vi "KE622x -- 2182 -A Get Params.vi"(0 "622x Resource In":refnum<visa-resource-name>, 1 "Check For SCPI Errors? (T)":bool=TRUE, 11 "error in (no error)":errorcluster) -> (4 "622x Resource Out (dupl)":refnum<visa-resource-name>, 8 "2182 -A Params":T1={"Auto Range?"=FALSE, "Man / Selected\n        Range"=0, "Enable Digital\n       Filter?"=FALSE, "Filter Type"=0, "Filter Count"=1, "      Filter\nWindow (%)"=0.01, "Enable Analog\n       Filter?"=FALSE, "NPLCs"=5} {"NPLCs" min=1 max=10; "Filter\nWindow (%)" min=0.01 max=10.0 step=0.01 format="%.2f"; "Filter Count" min=1 max=100; "Filter Type" items=["Movin", "Repeat"]; "Man / Selected\n        Range" items=["10mV", "100mV", "1V", "10V", "100V"]}, 15 "error out":errorcluster)   [LabVIEW 2013, in "Keithly user program.lvlib"]
uses:
  Keithly user program.lvlib
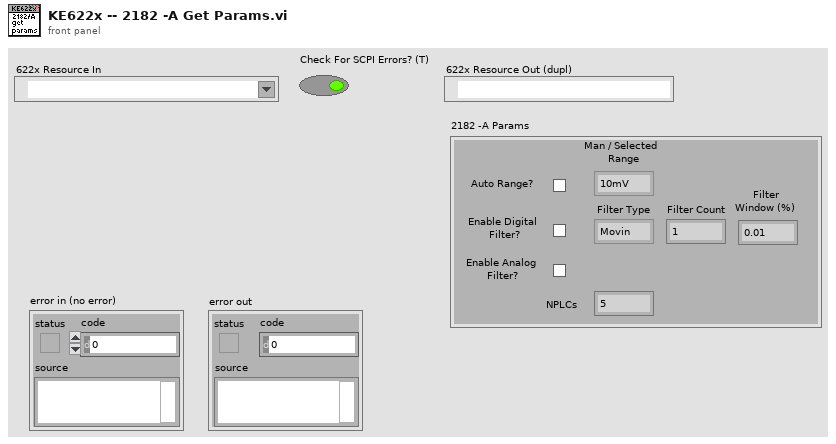
[diagram p1: front panel]
types:
  T1 = cluster{"Auto Range?":bool, "Man / Selected\n        Range":u16, "Enable Digital\n       Filter?":bool, "Filter Type":u16, "Filter Count":u32, "      Filter\nWindow (%)":dbl, "Enable Analog\n       Filter?":bool, "NPLCs":u32}
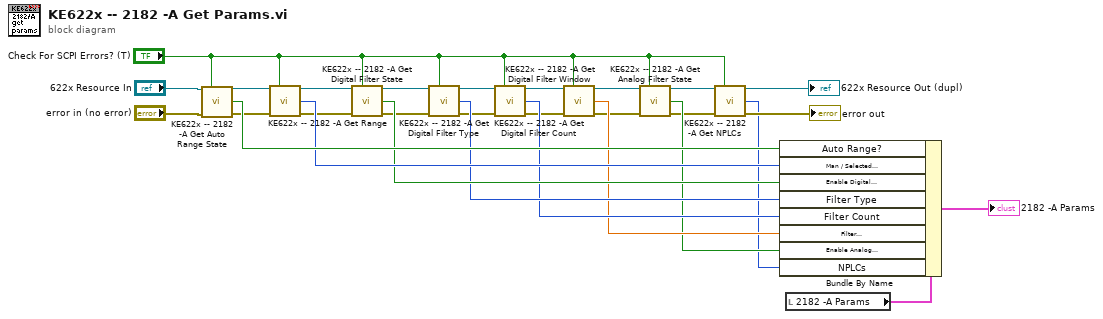
[diagram p0: block diagram]
diagram:
  n1 = call "KE622x -- 2182 -A Get Auto Range State.vi"("622x Resource In"="622x Resource In", "Check For SCPI Errors? (T)"="Check For SCPI Errors? (T)", "error in (no error)"="error in (no error)") -> ("622x Resource Out (dupl)"=w24:refnum<visa-resource-name>, "Auto Range Enabled?"=w25:bool, "error out"=w23:errorcluster)  [unwired: 10 in]
  n2 = call "KE622x -- 2182 -A Get Range.vi"("622x Resource In"=w24, "Check For SCPI Errors? (T)"="Check For SCPI Errors? (T)", "error in (no error)"=w23) -> ("622x Resource Out (dupl)"=w21:refnum<visa-resource-name>, "2182/2182A Range"=w22:enum16{"10mV", "100mV", "1V", "10V", "100V"}, "error out"=w20:errorcluster)  [unwired: 10 in]
  n3 = call "KE622x -- 2182 -A Get Digital Filter State.vi"("622x Resource In"=w21, "Check For SCPI Errors? (T)"="Check For SCPI Errors? (T)", "error in (no error)"=w20) -> ("622x Resource Out (dupl)"=w18:refnum<visa-resource-name>, "Digital Filter Enabled?"=w19:bool, "error out"=w17:errorcluster)  [unwired: 10 in]
  n4 = call "KE622x -- 2182 -A Get Digital Filter Type.vi"("622x Resource In"=w18, "Check For SCPI Errors? (T)"="Check For SCPI Errors? (T)", "error in (no error)"=w17) -> ("622x Resource Out (dupl)"=w15:refnum<visa-resource-name>, "Filter Type"=w16:enum16{"Movin", "Repeat"}, "error out"=w14:errorcluster)  [unwired: 10 in]
  n5 = call "KE622x -- 2182 -A Get Digital Filter Count.vi"("622x Resource In"=w15, "Check For SCPI Errors? (T)"="Check For SCPI Errors? (T)", "error in (no error)"=w14) -> ("622x Resource Out (dupl)"=w12:refnum<visa-resource-name>, "Filter Count"=w13:u32, "error out"=w11:errorcluster)  [unwired: 10 in]
  n6 = call "KE622x -- 2182 -A Get Digital Filter Window.vi"("622x Resource In"=w12, "Check For SCPI Errors? (T)"="Check For SCPI Errors? (T)", "error in (no error)"=w11) -> ("622x Resource Out (dupl)"=w9:refnum<visa-resource-name>, "Filter Window (%)"=w10:dbl, "error out"=w8:errorcluster)  [unwired: 10 in]
  n7 = call "KE622x -- 2182 -A Get Analog Filter State.vi"("622x Resource In"=w9, "Check For SCPI Errors? (T)"="Check For SCPI Errors? (T)", "error in (no error)"=w8) -> ("622x Resource Out (dupl)"=w5:refnum<visa-resource-name>, "Analog Filter Enabled?"=w7:bool, "error out"=w4:errorcluster)  [unwired: 10 in]
  n8 = call "KE622x -- 2182 -A Get NPLCs.vi"("622x Resource In"=w5, "Check For SCPI Errors? (T)"="Check For SCPI Errors? (T)", "error in (no error)"=w4) -> ("622x Resource Out (dupl)"=→"622x Resource Out (dupl)":refnum<visa-resource-name>, "2182 -A NPLCs 2"=w2:u32, "error out"=→"error out":errorcluster)  [unwired: 10 in]
  n9 = local read "2182 -A Params"() -> (w29:T1)
  n10 = Bundle By Name(cluster=w29, "Auto Range?"=w25, "Man / Selected\n        Range"=w22, "Enable Digital\n       Filter?"=w19, "Filter Type"=w16, "Filter Count"=w13, "Filter\nWindow (%)"=w10, "Enable Analog\n       Filter?"=w7, "NPLCs"=w2) -> (→"2182 -A Params":T1)
